vi "Draw Line.vi"(6 "Colour":u32(colorbox), 9 "Point 2":T1, 10 "Point 1":T1, 11 "Pixel Data in":u32[][](array[numeric])) -> (3 "Pixel Data out":u32[][](array[numeric]))   [LabVIEW 2022 SP3, in "Raster.lvlib"]
uses:
  Raster.lvlib
  Point 2D.ctl
  <vilib>/Utility/High Resolution Relative Seconds.vi
  Utility/Utility.lvlib
panel:
  out "Processing Time [s]":dbl format="%.1p"
  out "Iteration":i32
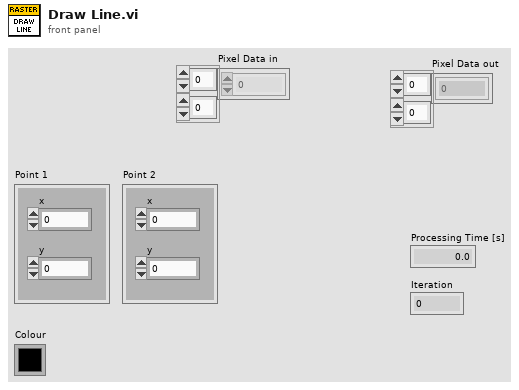
[diagram p1: front panel]
types:
  T1 = typedef "Raster.lvlib/Point 2D.ctl" = cluster{"x":i32, "y":i32}
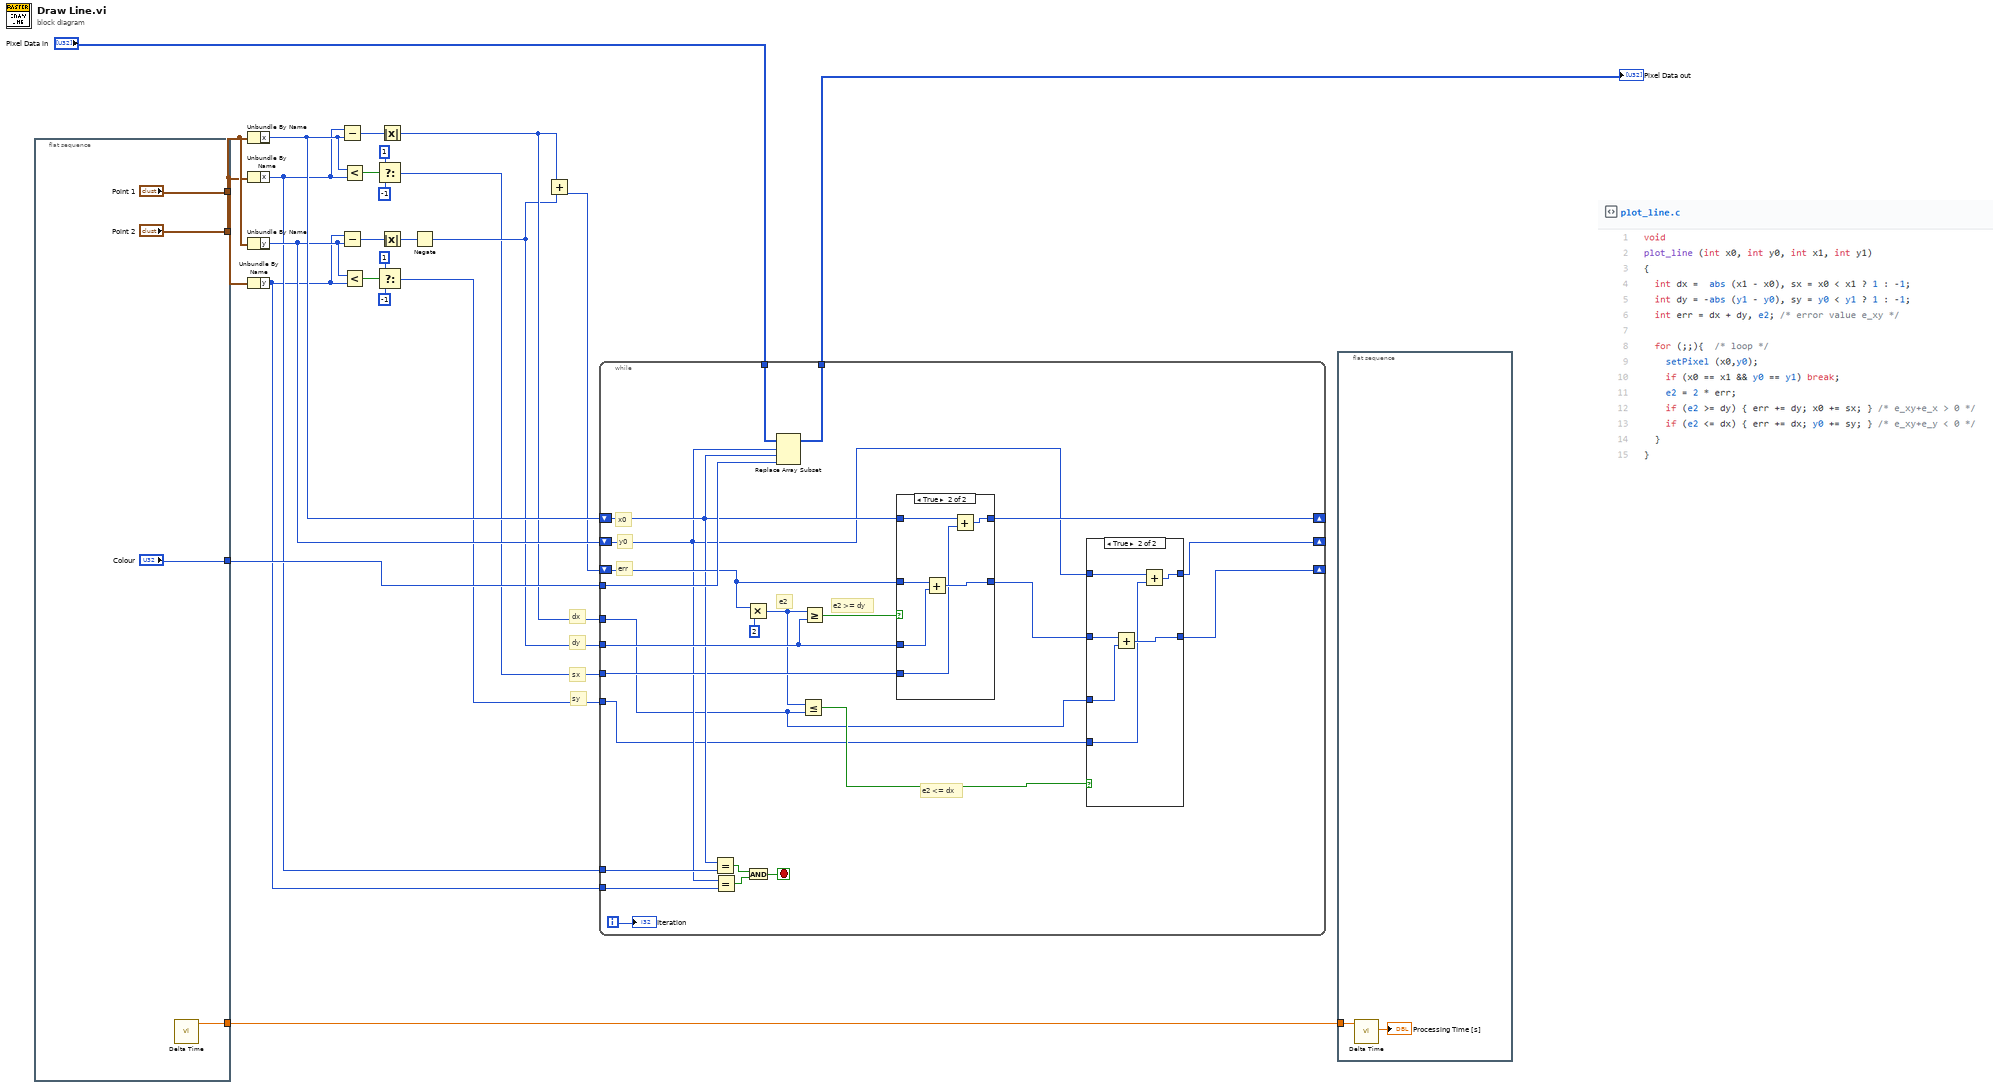
[diagram p0: block diagram]
diagram:
  # "sy"
  # "sx"
  # "dy"
  # "dx"
  n1 = flat-sequence {
    tunnel: ["Point 1"] -> w16
    tunnel: ["Point 2"] -> w15
    tunnel: ["Colour"] -> w11
    tunnel: [w25] -> w3
    frame #0 {
      n2 = call "Delta Time.vi"() -> ("Relative Seconds Out"=w25:dbl)  [unwired: 10 in, 1 out]
    }
  }
  n3 = Unbundle By Name(w16) -> ("x"=w13:i32)
  n4 = Unbundle By Name(w15) -> ("x"=w10:i32)
  n5 = Unbundle By Name(w16) -> ("y"=w12:i32)
  n6 = Unbundle By Name(w15) -> ("y"=w9:i32)
  n7 = Subtract(x=w10, y=w13) -> (x-y=w24:i32)
  n8 = Subtract(x=w9, y=w12) -> (x-y=w17:i32)
  n9 = Less?(x=w13, y=w10) -> (x < y?=w23:bool)
  n10 = Less?(x=w12, y=w9) -> (x < y?=w18:bool)
  n11 = Select(t=1 ("x-y"), s=w23, f=-1 ("x-y")) -> (s? t:f=w5:i32)
  n12 = Select(t=1 ("x-y"), s=w18, f=-1 ("x-y")) -> (s? t:f=w4:i32)
  n13 = Absolute Value(x=w24) -> (abs(x)=w7:i32)
  n14 = Absolute Value(x=w17) -> (abs(x)=w14:i32)
  n15 = Negate(x=w14) -> (-x=w6:i32)
  n16 = Add(x=w7, y=w6) -> (x+y=w8:i32)
  n17 = while {
    shift-right: [w40] -> _
    shift-left: w13 -> [w42]
    shift-right: [w35] -> _
    shift-left: w12 -> [w36]
    tunnel: w11 -> [w52]
    tunnel: w10 -> [w51]
    tunnel: w9 -> [w50]
    shift-right: [w33] -> _
    shift-left: w8 -> [w44]
    tunnel: w7 -> [w34]
    tunnel: w6 -> [w43]
    tunnel: w5 -> [w41]
    tunnel: w4 -> [w32]
    tunnel: "Pixel Data in" -> [w30]
    tunnel: [w29] -> w1
    i -> [w31]
    stop <- w47 stop-if-true
    # "e2 <= dx"
    # "e2 >= dy"
    # "e2"
    # "err"
    # "y0"
    # "x0"
    n18 = Equal?(x=w42, y=w51) -> (x = y?=w49:bool)
    n19 = Equal?(x=w36, y=w50) -> (x = y?=w48:bool)
    n20 = Multiply(x=w44, y=2) -> (x*y=w39:i32)
    n21 = And(x=w49, y=w48) -> (x .and. y?=w47:bool)
    n22 = Replace Array Subset(array=w30, new element=w52, index (row)=w36, index (col)=w42) -> (w29:u32[][])
    n23 = Less Or Equal?(x=w39, y=w34) -> (x <= y?=w38:bool)
    n24 = Greater Or Equal?(x=w39, y=w43) -> (x >= y?=w45:bool)
    n25 = case shown="True" w45 {
      tunnel: w44 -> [w53 w60]
      tunnel: w43 -> [_ w59]
      tunnel: [w53 w58] -> w37
      tunnel: w42 -> [w54 w57]
      tunnel: w41 -> [_ w56]
      tunnel: [w54 w55] -> w40
      frame False {
      }
      frame True {
        n26 = Add(x=w60, y=w59) -> (x+y=w58:i32)
        n27 = Add(x=w57, y=w56) -> (x+y=w55:i32)
      }
    }
    n28 = case shown="True" w38 {
      tunnel: w37 -> [w62 w68]
      tunnel: w34 -> [_ w67]
      tunnel: [w62 w66] -> w33
      tunnel: w36 -> [w61 w65]
      tunnel: w32 -> [_ w64]
      tunnel: [w61 w63] -> w35
      frame False {
      }
      frame True {
        n29 = Add(x=w68, y=w67) -> (x+y=w66:i32)
        n30 = Add(x=w65, y=w64) -> (x+y=w63:i32)
      }
    }
    "Iteration" <- w31
  }
  "Pixel Data out" <- w1
  n31 = flat-sequence {
    tunnel: w3 -> [w70]
    frame #0 {
      n32 = call "Delta Time.vi"("Relative Seconds In"=w70) -> ("Delta Time [s]"=→"Processing Time [s]":dbl)  [unwired: 9 in, 1 out]
    }
  }
